vi "loop_generated_array.vi"() -> ()   [LabVIEW 2019]
panel:
  out "Array 4":i32[](array[numeric])
  out "Array 3":i32[][](array[numeric])
  out "Array 2":i32[](array[numeric])
  out "Numeric":i32
  out "Array":i32[](array[numeric])
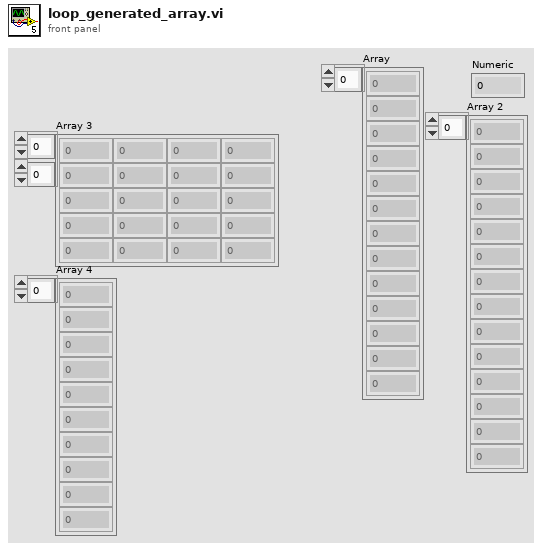
[diagram p1: front panel]
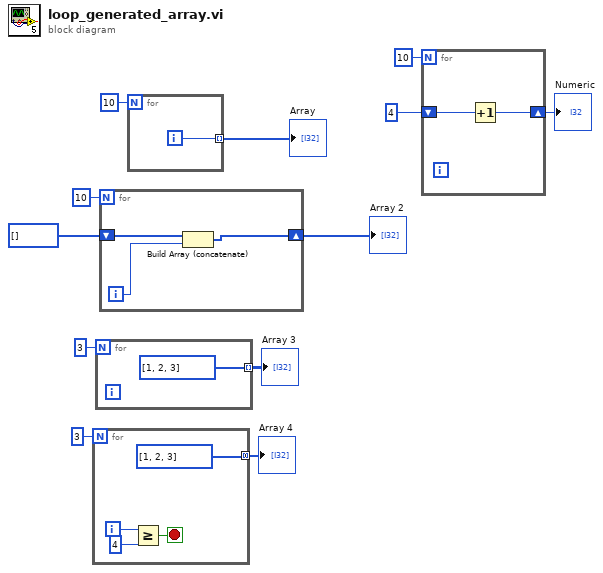
[diagram p0: block diagram]
diagram:
  n1 = for {
    N: 3 -> [_]
    tunnel: [i32[] [1, 2, 3]] -> w1 mode=concatenating
    i -> [w15]
    stop <- w13 stop-if-true
    n2 = Greater Or Equal?(x=w15, y=4) -> (x >= y?=w13:bool)
  }
  "Array 4" <- w1
  n3 = for {
    N: 3 -> [_]
    tunnel: [i32[] [1, 2, 3]] -> w3 mode=indexing
  }
  "Array 3" <- w3
  n4 = for {
    N: 10 -> [_]
    shift-right: [w18] -> w5
    shift-left: i32[] [] -> [w20]
    i -> [w19]
    n5 = Build Array (concatenate)(w20, w19) -> (w18:i32[])
  }
  "Array 2" <- w5
  n6 = for {
    N: 10 -> [_]
    tunnel: [w21] -> w11 mode=indexing
    i -> [w21]
  }
  "Array" <- w11
  n7 = for {
    N: 10 -> [_]
    shift-right: [w22] -> w8
    shift-left: 4 -> [w23]
    n8 = Increment(x=w23) -> (x+1=w22:i32)
  }
  "Numeric" <- w8
